vi "HardwareLoop.vi"(8 "Error In":errorcluster, 10 "Data Structures":T1, 11 "Action Queues":T2) -> (0 "Error Out":errorcluster)   [LabVIEW 2012]
uses:
  ActionQueues.ctl
  UIActionQueueElement.ctl
  UIAction.ctl
  HardwareActionQueueElement.ctl
  HardwareAction.ctl
  HeaterActionQueueElement.ctl
  HeaterAction.ctl
  MFCActionQueueElement.ctl
  MFCAction.ctl
  LogActionQueueElement.ctl
  LogAction.ctl
  DataStructures.ctl
  HardwareDisplayData.ctl
  HardwareLogData.ctl
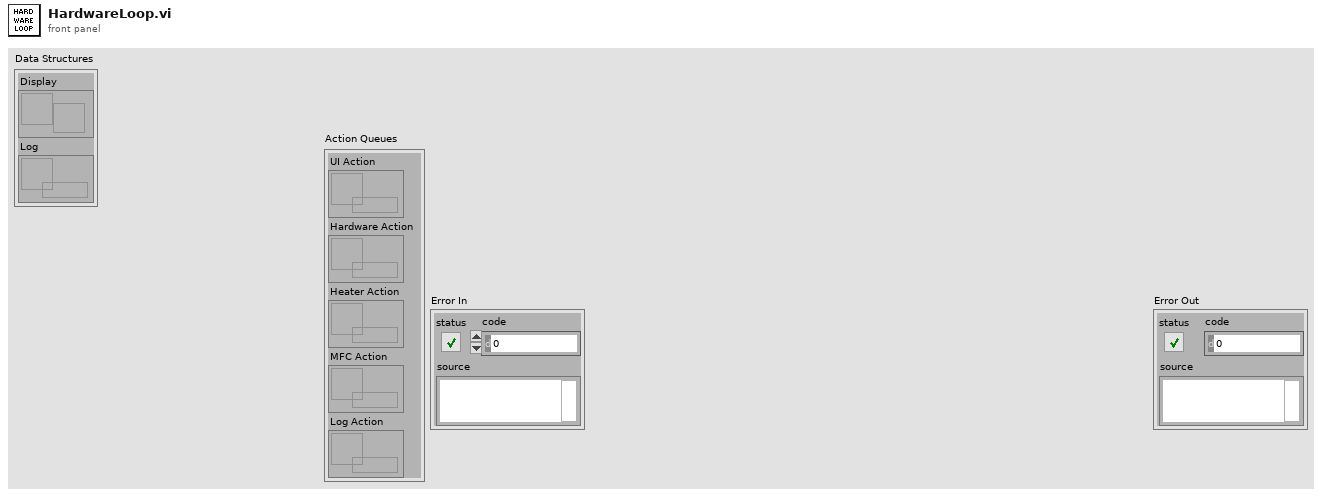
[diagram p1: front panel]
types:
  T1 = typedef "DataStructures.ctl" = cluster{"Display":refnum<notifier>, "Log":refnum<queue>}
  T2 = typedef "ActionQueues.ctl" = cluster{"UI Action":refnum<queue>, "Hardware Action":refnum<queue>, "Heater Action":refnum<queue>, "MFC Action":refnum<queue>, "Log Action":refnum<queue>}
  T3 = typedef "HardwareDataStructures.ctl" = cluster{"Heater":refnum<notifier>, "MFC":refnum<notifier>}
  T4 = typedef "HardwareDisplayData.ctl" = cluster{"Heater":dbl, "MFC":dbl}
  T5 = typedef "HardwareLogData.ctl" = cluster{"Timestamp":timestamp, "Data":T4}
  T6 = typedef "HardwareActionQueueElement.ctl" = cluster{"Action":T7, "Data":variant}
  T7 = typedef "HardwareAction.ctl" = enum16{"Initialize", "Collect", "Shutdown"}
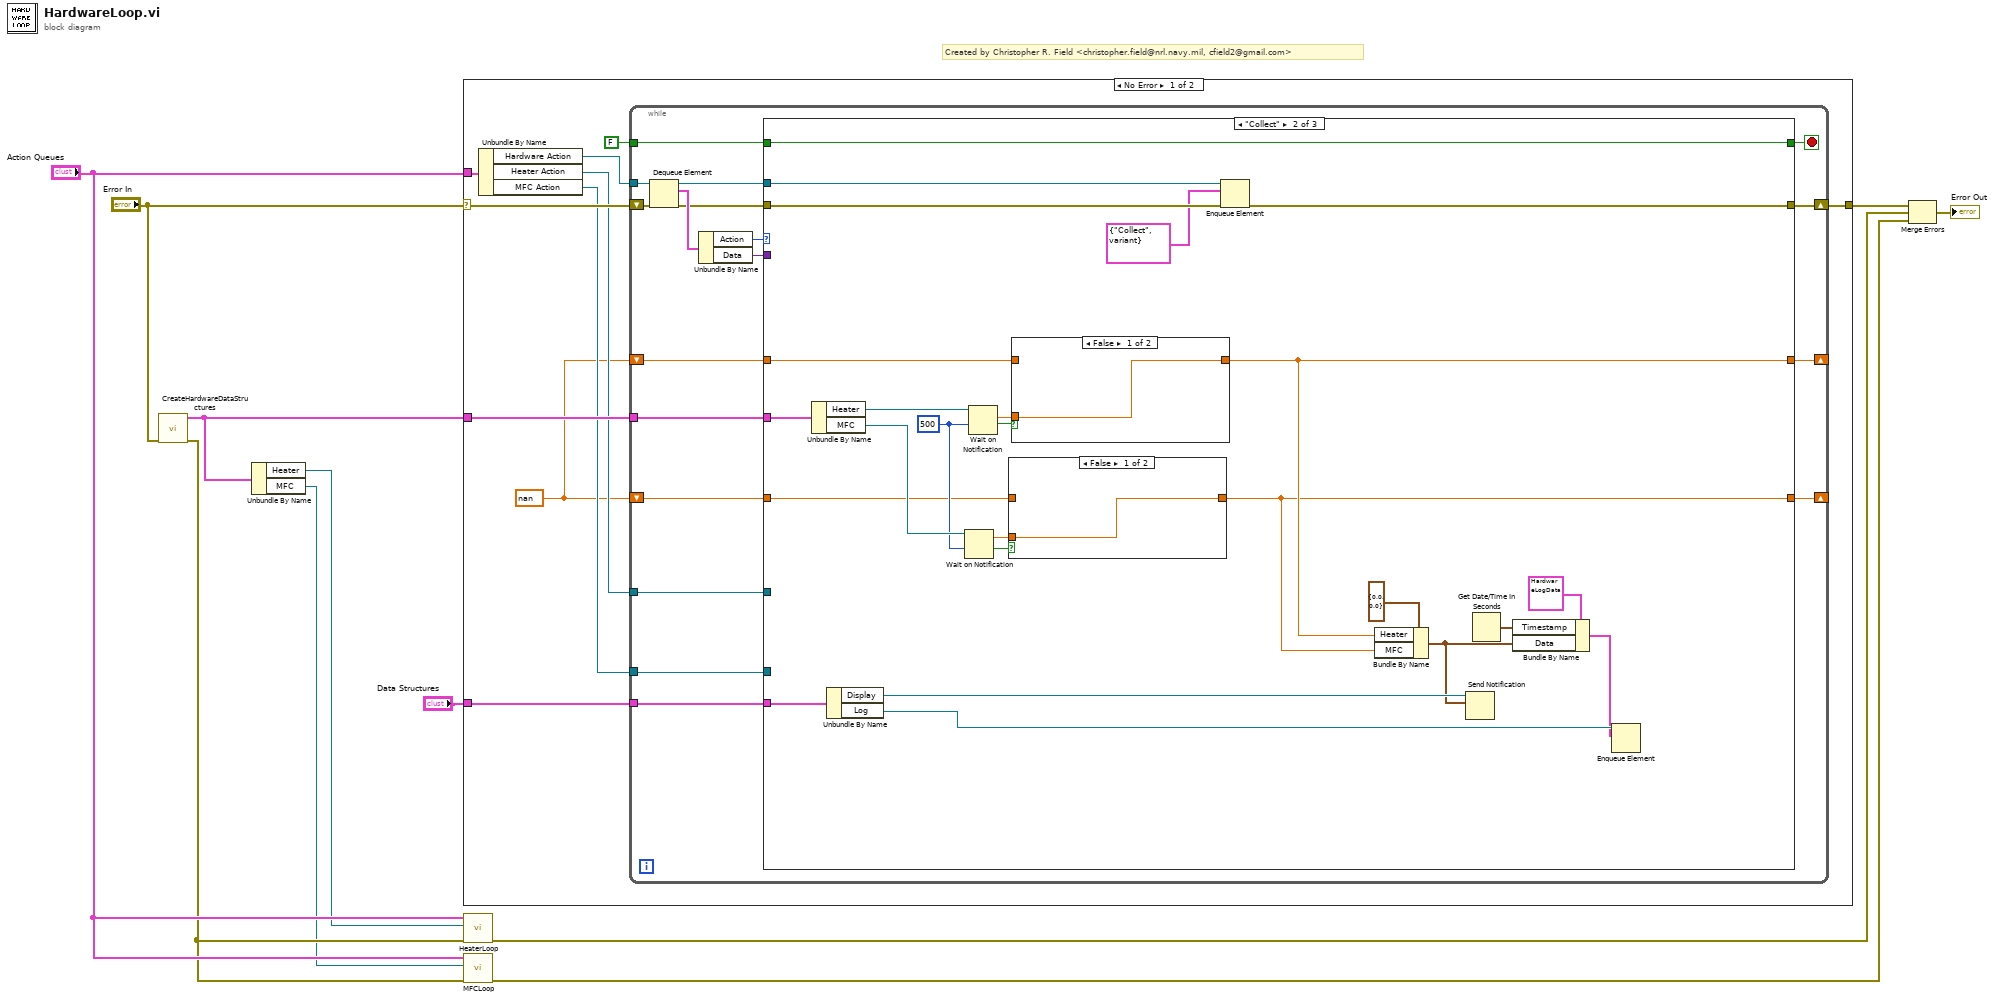
[diagram p0: block diagram]
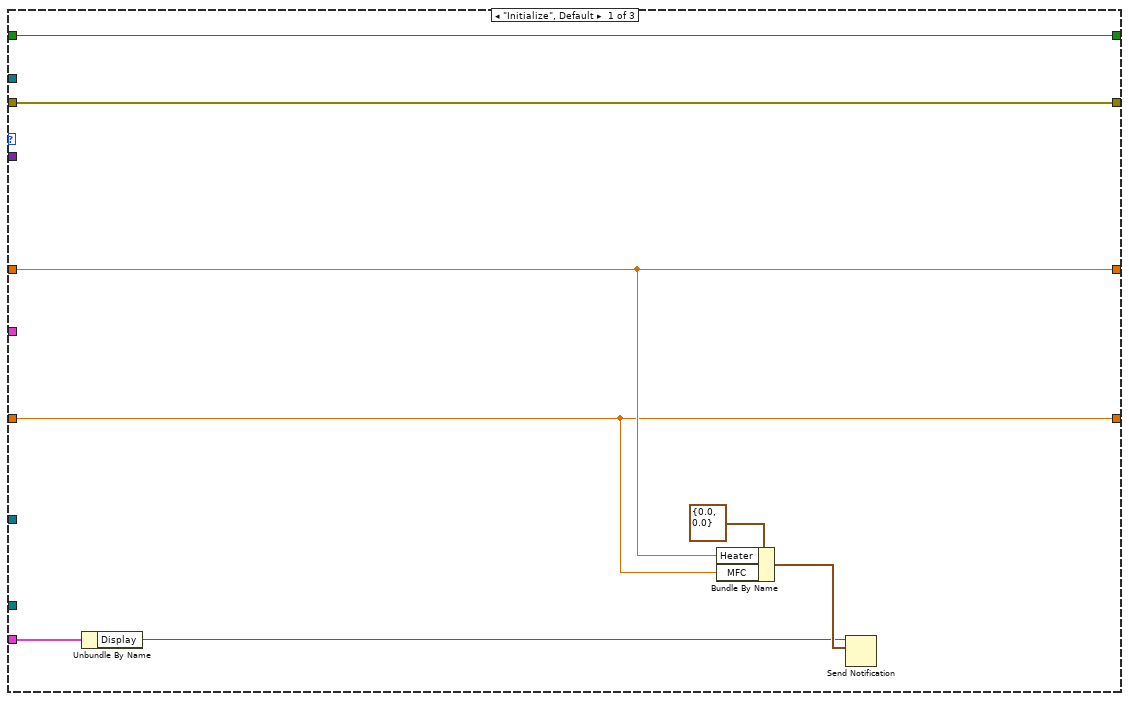
[diagram p2: hidden frame]
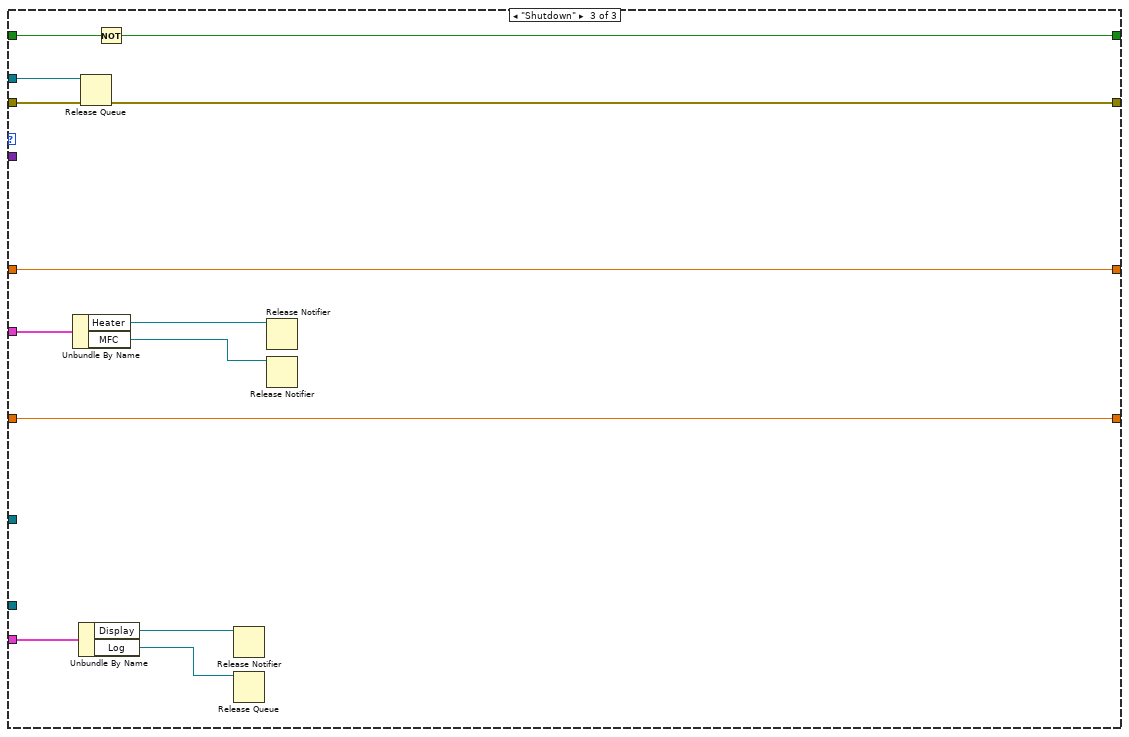
[diagram p5: hidden frame]
diagram:
  # "Created by Christopher R. Field <christopher.field@nrl.navy.mil, cfield2@gmail.com>"
  n1 = call "CreateHardwareDataStructures.vi"("Error In"="Error In") -> ("Error Out"=w3:errorcluster, "Hardware Data Structures"=w6:T3)  [unwired: 9 in]
  n2 = Unbundle By Name(w6) -> ("Heater"=w1:refnum<notifier>, "MFC"=w2:refnum<notifier>)
  n3 = case shown="No Error" "Error In" {
    selector: "Error In" -> [w17 w90]
    tunnel: [w20 w90] -> w11
    tunnel: "Action Queues" -> [w19 _]
    tunnel: "Data Structures" -> [w16 _]
    tunnel: w6 -> [w15 _]
    frame No Error {
      w12 = nan
      n4 = Unbundle By Name(w19) -> ("Hardware Action"=w18:refnum<queue>, "Heater Action"=w14:refnum<queue>, "MFC Action"=w13:refnum<queue>)
      n5 = while {
        tunnel: FALSE -> [w39]
        shift-right: [w32] -> w20
        shift-left: w17 -> [w38]
        tunnel: w18 -> [w30]
        tunnel: w15 -> [w29]
        tunnel: w16 -> [w28]
        tunnel: w14 -> [w27]
        tunnel: w13 -> [w26]
        shift-right: [w25] -> _
        shift-left: w12 -> [w24]
        shift-right: [w22] -> _
        shift-left: w12 -> [w23]
        stop <- w31 stop-if-true
        n6 = Dequeue Element(queue=w30, error in (no error)=w38) -> (queue out=w37:refnum<queue>, element=w36:T6, error out=w33:errorcluster)  [unwired: 1 in, 1 out]
        n7 = Unbundle By Name(w36) -> ("Action"=w35:T7, "Data"=w34:variant)
        n8 = case shown="\"Collect\"" w35 {
          tunnel: w39 -> [w47 w72 w89]
          tunnel: w37 -> [_ w71 w87]
          tunnel: w34 -> [_ _ _]
          tunnel: w33 -> [w46 w70 w86]
          tunnel: [w46 w69 w85] -> w32
          tunnel: [w47 w72 w88] -> w31
          tunnel: w29 -> [_ w66 w82]
          tunnel: w28 -> [w45 w58 w84]
          tunnel: w27 -> [_ _ _]
          tunnel: w26 -> [_ _ _]
          tunnel: [w40 w48 w77] -> w25
          tunnel: w24 -> [w40 w51 w77]
          tunnel: w23 -> [w41 w50 w78]
          tunnel: [w41 w49 w78] -> w22
          frame "Initialize", Default {
            n9 = Unbundle By Name(w45) -> ("Display"=w42:refnum<notifier>)
            n10 = Bundle By Name(cluster=T4 {"Heater"=0.0, "MFC"=0.0} ("Hardware Display Data"), "Heater"=w41, "MFC"=w40) -> (w43:T4)
            n11 = Send Notification(notification=w43, notifier=w42) -> ()  [unwired: 1 in, 2 out]
          }
          frame "Collect" {
            w60 = 500 ("timeout in ms (-1)")
            n12 = Unbundle By Name(w66) -> ("Heater"=w65:refnum<notifier>, "MFC"=w64:refnum<notifier>)
            n13 = Unbundle By Name(w58) -> ("Display"=w57:refnum<notifier>, "Log"=w56:refnum<queue>)
            n14 = Wait on Notification(notifier=w64, timeout in ms (-1)=w60) -> (notification=w61:dbl, timed out?=w62:bool)  [unwired: 2 in, 2 out]
            n15 = Wait on Notification(notifier=w65, timeout in ms (-1)=w60) -> (notification=w63:dbl, timed out?=w67:bool)  [unwired: 2 in, 2 out]
            n16 = case shown="False" w62 {
              tunnel: w61 -> [w73 _]
              tunnel: [w73 w74] -> w48
              tunnel: w51 -> [_ w74]
              frame False {
              }
              frame True {
              }
            }
            n17 = case shown="False" w67 {
              tunnel: w63 -> [w75 _]
              tunnel: w50 -> [_ w76]
              tunnel: [w75 w76] -> w49
              frame False {
              }
              frame True {
              }
            }
            n18 = Enqueue Element(queue=w71, element=T6 {"Action"=enum."Collect", "Data"=variant}, error in (no error)=w70) -> (error out=w69:errorcluster)  [unwired: 1 in, 2 out]
            n19 = Bundle By Name(cluster=T4 {"Heater"=0.0, "MFC"=0.0} ("Hardware Display Data"), "Heater"=w49, "MFC"=w48) -> (w53:T4)
            n20 = Send Notification(notification=w53, notifier=w57) -> ()  [unwired: 1 in, 2 out]
            n21 = Get Date/Time In Seconds() -> (seconds since 1Jan1904=w54:timestamp)
            n22 = Bundle By Name(cluster=T5 {"Timestamp"=timestamp(0 s since 1904-01-01), "Data"={"Heater"=0.0, "MFC"=0.0}} ("Hardware Log Data"), "Timestamp"=w54, "Data"=w53) -> (w52:T5)
            n23 = Enqueue Element(queue=w56, element=w52) -> ()  [unwired: 2 in, 3 out]
          }
          frame "Shutdown" {
            n24 = Unbundle By Name(w82) -> ("Heater"=w81:refnum<notifier>, "MFC"=w80:refnum<notifier>)
            n25 = Unbundle By Name(w84) -> ("Display"=w83:refnum<notifier>, "Log"=w79:refnum<queue>)
            n26 = Release Queue(queue=w87, error in (no error)=w86) -> (error out=w85:errorcluster)  [unwired: 1 in, 2 out]
            n27 = Not(x=w89) -> (.not. x?=w88:bool)
            n28 = Release Notifier(notifier=w83) -> ()  [unwired: 2 in, 3 out]
            n29 = Release Queue(queue=w79) -> ()  [unwired: 2 in, 3 out]
            n30 = Release Notifier(notifier=w81) -> ()  [unwired: 2 in, 3 out]
            n31 = Release Notifier(notifier=w80) -> ()  [unwired: 2 in, 3 out]
          }
        }
      }
    }
    frame Error {
    }
  }
  n32 = call "HeaterLoop.vi"("Error In"=w3, "Heater Data"=w1, "Action Queues"="Action Queues") -> ("Error Out"=w8:errorcluster)  [unwired: 8 in]
  n33 = call "MFCLoop.vi"("Error In"=w3, "MFC Data"=w2, "Action Queues"="Action Queues") -> ("Error Out"=w7:errorcluster)  [unwired: 8 in]
  n34 = Merge Errors(w11, w8, w7) -> (→"Error Out":errorcluster)
